vi "_Measure 1 Period.vi"() -> ()   [LabVIEW 2014]
panel:
  out "number of samples":dbl
  out "in":u16[](graph)
  out "out":u16[](graph)
  out "tmr 2 rld value":u16
  in  "Signal freq [Hz]":u32
  in  "VISA resource name":refnum<visa-resource-name>
  out "VISA Refnum out 2":refnum<visa-resource-name>
  out "error out 2":errorcluster
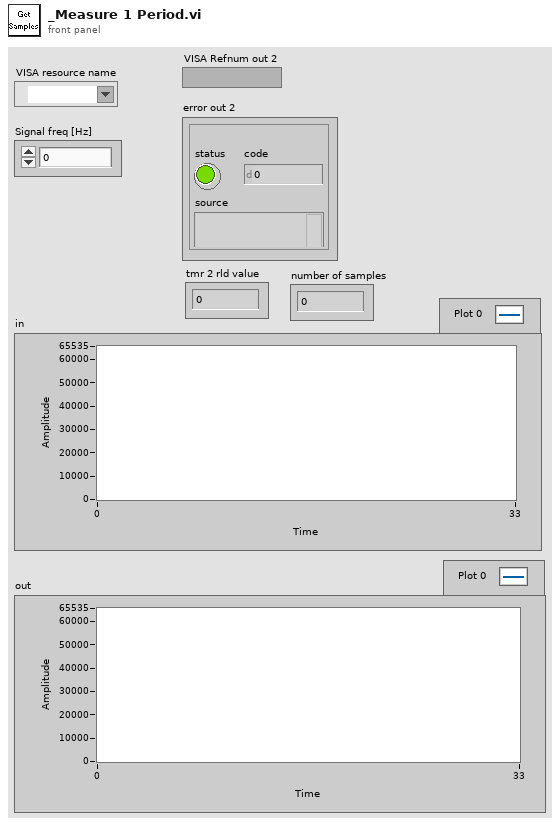
[diagram p1: front panel]
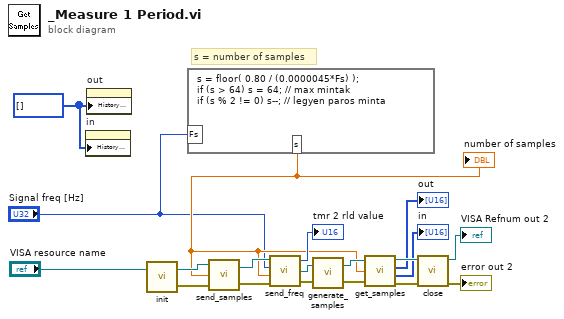
[diagram p0: block diagram]
diagram:
  w2 = u16[] [] ("History Data")
  # "s = number of samples"
  n1 = property on="in" class="WFChart (strict)"("History Data"=w2) -> ()  [unwired: 2 in, 2 out]
  n2 = property on="out" class="WFChart (strict)"("History Data"=w2) -> ()  [unwired: 2 in, 2 out]
  n3 = call "init.vi"("VISA Refnum in"="VISA resource name") -> ("error out"=w11:errorcluster, "VISA Refnum out"=w12:refnum<visa-resource-name>)  [unwired: 1 in]
  n4 = formula code="s = floor( 0.80 / (0.0000045*Fs) );\nif (s > 64) s = 64; // max mintak\nif (s % 2 != 0) s--; // legyen paros minta"("Fs"="Signal freq [Hz]") -> ("s"=w3:dbl)
  "number of samples" <- w3
  n5 = call "send_samples.vi"("error in (no error)"=w11, "elemszam"=w3, "VISA Refnum in"=w12) -> ("error out"=w9:errorcluster, "VISA Refnum out"=w10:refnum<visa-resource-name>)
  n6 = call "send_freq.vi"("error in (no error)"=w9, "elemszam"=w3, "signal freq"="Signal freq [Hz]", "VISA Refnum in"=w10) -> ("error out"=w8:errorcluster, "VISA Refnum out"=w6:refnum<visa-resource-name>, "tmr 2 rld value"=→"tmr 2 rld value":u16)
  n7 = call "generate_samples.vi"("error in (no error)"=w8, "VISA Refnum in"=w6) -> ("error out"=w15:errorcluster, "VISA Refnum out"=w16:refnum<visa-resource-name>)
  n8 = call "get_samples.vi"("VISA Refnum in"=w16, "#Samples to read"=w3, "error in (no error)"=w15) -> ("VISA Refnum out"=w14:refnum<visa-resource-name>, "out samples"=→"out":u16[], "in samples"=→"in":u16[], "error out"=w13:errorcluster)
  n9 = call "close.vi"("error in (no error)"=w13, "VISA resource name"=w14) -> ("error out"=→"error out 2":errorcluster, "VISA resource name out"=→"VISA Refnum out 2":refnum<visa-resource-name>)  [unwired: 4 in]
